vi "Get image.vi"(8 "error in (no error)":errorcluster, 11 "CCD in":refnum<class "CCD.lvclass">) -> (0 "error out":errorcluster, 3 "CCD out":refnum<class "CCD.lvclass">)   [LabVIEW 2018, in "CCD.lvclass"]
uses:
  CCD.lvclass
  CCD.lvclass/CCD.ctl
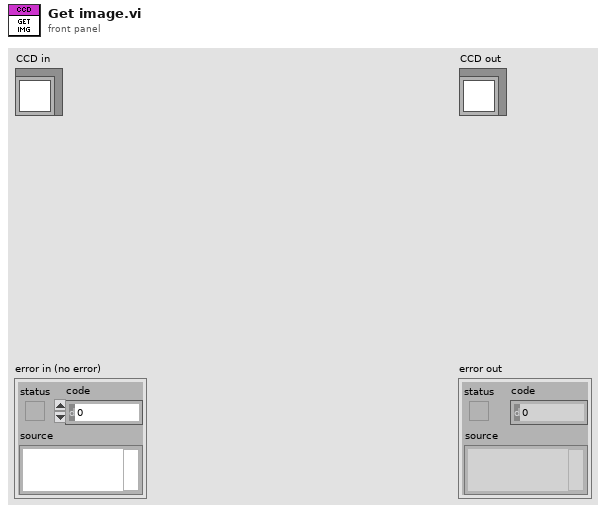
[diagram p1: front panel]
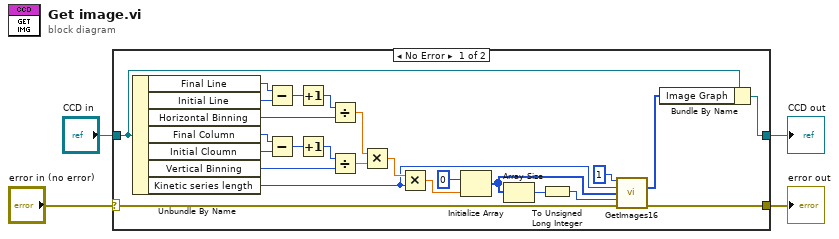
[diagram p0: block diagram]
diagram:
  n1 = case shown="No Error" "error in (no error)" {
    selector: "error in (no error)" -> [w11 w31]
    tunnel: [w6 w31] -> w3
    tunnel: [w7 w30] -> w1
    tunnel: "CCD in" -> [w9 w30]
    frame No Error {
      n2 = Unbundle By Name(w9) -> ("Final Line"=w17:u16, "Initial Line"=w16:u16, "Horizontal Binning"=w15:u16, "Final Column"=w14:u16, "Initial Cloumn"=w13:u16, "Vertical Binning"=w12:u16, "Kinetic series length"=w5:u32)
      n3 = Subtract(x=w17, y=w16) -> (x-y=w28:u16)
      n4 = Subtract(x=w14, y=w13) -> (x-y=w27:u16)
      n5 = Increment(x=w28) -> (x+1=w29:u16)
      n6 = Increment(x=w27) -> (x+1=w25:u16)
      n7 = Divide(x=w29, y=w15) -> (x/y=w26:dbl)
      n8 = Divide(x=w25, y=w12) -> (x/y=w24:dbl)
      n9 = Multiply(x=w26, y=w24) -> (x*y=w23:dbl)
      n10 = Multiply(x=w23, y=w5) -> (x*y=w20:dbl)
      n11 = Initialize Array(u16 0, w20) -> (w18:u16[])
      n12 = Array Size(array=w18) -> (size(s)=w22:i32)
      n13 = To Unsigned Long Integer(number=w22) -> (unsigned 32bit integer=w21:u32)
      n14 = call <userlib>:"GetImages16.vi"("first"=1, "last"=w5, "array"=w18, "size"=w21, "error in (no error)"=w11) -> ("array"=w8:u16[], "error out"=w6:errorcluster)  [unwired: 6 in, 3 out]
      n15 = Bundle By Name(cluster=w9, "Image Graph"=w8) -> (w7:refnum<class "CCD.lvclass">)
    }
    frame Error {
    }
  }
  "error out" <- w3
  "CCD out" <- w1
